vi "ConvertTo(path).vi"(8 "error in":errorcluster, 9 "Message Payload":variant) -> (0 "error out":errorcluster, 1 "Message Payload path":path)   [LabVIEW 2017]
doc: "Convert variant to path\n\nBolder Software LLC"
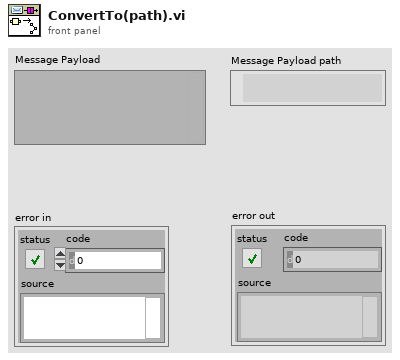
[diagram p1: front panel]
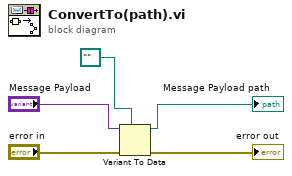
[diagram p0: block diagram]
diagram:
  n1 = Variant To Data(error in="error in", type=path "" ("Message Payload error"), Variant="Message Payload") -> (data=→"Message Payload path":path, error out=→"error out":errorcluster)
